vi "Refnums.vi"() -> ()   [LabVIEW 2015]
panel:
  in  "Gunner":string="Gunner"
  in  "Drive":string="Drive"
  in  "Left1":string="Left1"
  in  "Left2":string="Left2"
  in  "Left3":string="Left3"
  in  "Right3":string="Right3"
  in  "Right1":string="Right1"
  in  "Right2":string="Right2"
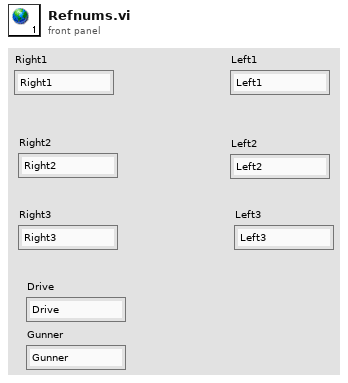
[diagram p1: front panel]
diagram:
